vi "Configure Exposure.vi"(8 "error in (no error)":errorcluster, 10 "exposure":u32, 11 "TroSpec in":refnum<class "PL ISTEQ TroSpec.lvclass">) -> (0 "error out":errorcluster, 3 "TroSpec out":refnum<class "PL ISTEQ TroSpec.lvclass">)   [LabVIEW 2015, in "PL ISTEQ TroSpec.lvclass"]
doc: "Configures exposure."
uses:
  PL ISTEQ TroSpec.lvclass
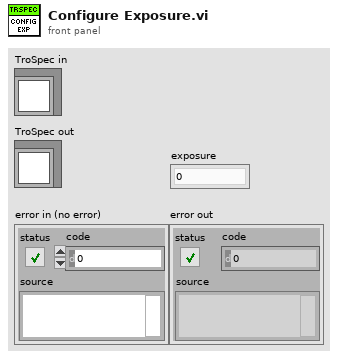
[diagram p1: front panel]
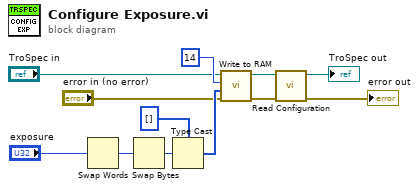
[diagram p0: block diagram]
diagram:
  n1 = Swap Words(1:"exposure") -> (0:w5:u32)
  n2 = Swap Bytes(anything=w5) -> (byte swapped=w7:u32)
  n3 = Type Cast(type=u8[] [] ("data"), x=w7) -> (*(type *) &x=w12:u8[])
  n4 = call "Write to RAM.vi"("error in (no error)"="error in (no error)", "data"=w12, "address"=u16 14, "TroSpec in"="TroSpec in") -> ("error out"=w3:errorcluster, "TroSpec out"=w4:refnum<class "PL ISTEQ TroSpec.lvclass">)  [unwired: 6 in]
  n5 = call "Read Configuration.vi"("error in (no error)"=w3, "TroSpec in"=w4) -> ("error out"=→"error out":errorcluster, "TroSpec out"=→"TroSpec out":refnum<class "PL ISTEQ TroSpec.lvclass">)  [unwired: 7 in, 1 out]
